vi "subMooseAlgorithm.vi"(0 "input":cdb[](array[numeric]), 5 "Training Sequence":cdb[](array[numeric]), 9 "symbol rate":dbl, 11 "channel estimate length":i32, 12 "Correct Frequency Offset?":bool=TRUE) -> (4 "output":cdb[](array[numeric]), 15 "frequency offset (Hz)":dbl)   [LabVIEW 2011]
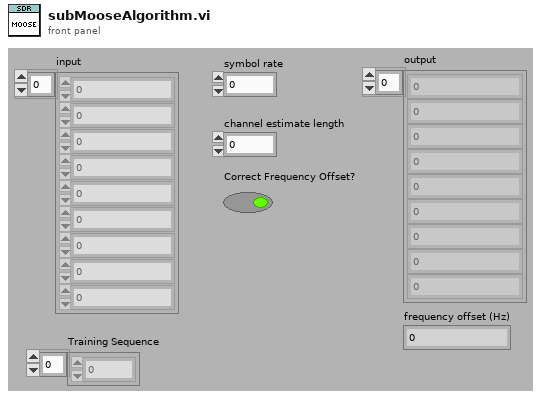
[diagram p1: front panel]
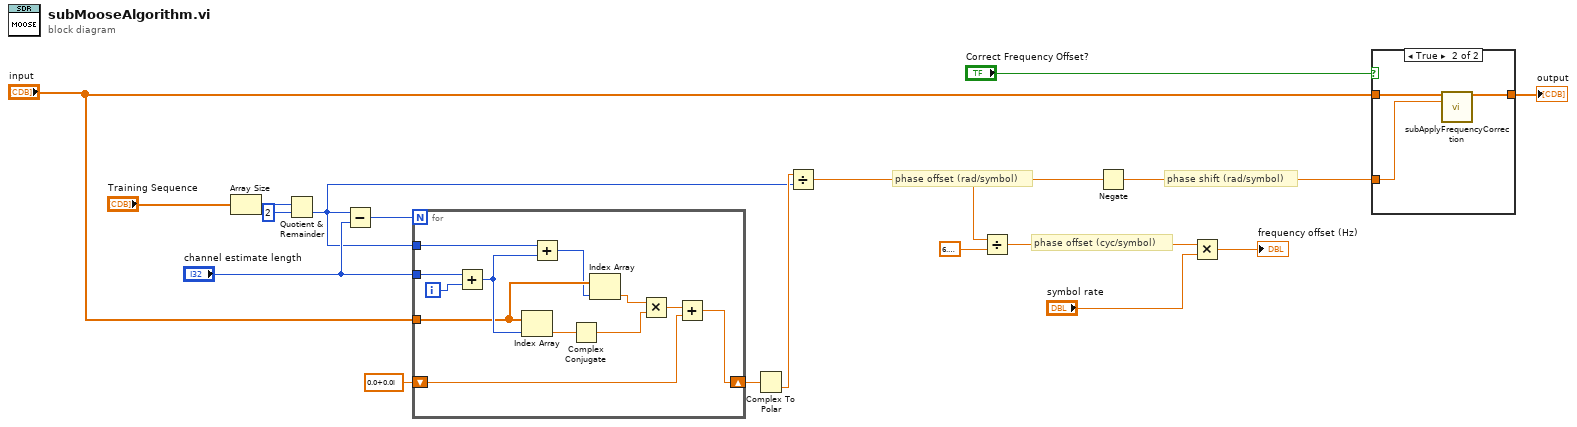
[diagram p0: block diagram]
diagram:
  # "phase offset (rad/symbol)"
  # "phase shift (rad/symbol)"
  # "phase offset (cyc/symbol)"
  n1 = Array Size(array="Training Sequence") -> (size(s)=w18:i32)
  n2 = Quotient & Remainder(x=w18, y=2) -> (floor(x/y)=w5:i32)  [unwired: 1 out]
  n3 = Subtract(x=w5, y="channel estimate length") -> (x-y=w6:i32)
  n4 = for {
    N: w6 -> [_]
    tunnel: "input" -> [w25]
    tunnel: "channel estimate length" -> [w29]
    tunnel: w5 -> [w28]
    shift-right: [w20] -> w14
    shift-left: cdb 0.0+0.0i -> [w19]
    i -> [w30]
    n5 = Add(x=w29, y=w30) -> (x+y=w27:i32)
    n6 = Index Array(array=w25, index=w27) -> (element=w26:cdb)
    n7 = Add(x=w28, y=w27) -> (x+y=w24:i32)
    n8 = Complex Conjugate(1:w26) -> (0:w22:cdb)
    n9 = Index Array(array=w25, index=w24) -> (element=w23:cdb)
    n10 = Multiply(x=w23, y=w22) -> (x*y=w21:cdb)
    n11 = Add(x=w21, y=w19) -> (x+y=w20:cdb)
  }
  n12 = Complex To Polar(r * e^(i*theta)=w14) -> (theta=w13:dbl)  [unwired: 1 out]
  n13 = Divide(x=w13, y=w5) -> (x/y=w3:dbl)
  n14 = Divide(x=w3, y=6.283185307179586) -> (x/y=w2:dbl)
  n15 = Negate(x=w3) -> (-x=w1:dbl)
  n16 = Multiply(x=w2, y="symbol rate") -> (x*y=→"frequency offset (Hz)":dbl)
  n17 = case shown="True" "Correct Frequency Offset?" {
    tunnel: "input" -> [w31 w34]
    tunnel: w1 -> [_ w33]
    tunnel: [w31 w32] -> w9
    frame False {
    }
    frame True {
      n18 = call "subApplyFrequencyCorrection.vi"("input signal"=w34, "phase shift (rad/point)"=w33) -> ("output signal"=w32:cdb[])  [unwired: 12 in, 1 out]
    }
  }
  "output" <- w9
